vi "Accept UDP command logic.vi"(9 "Msg in":T1, 10 "MC IP":string, 11 "Msg in 2":T1) -> (2 "Boolean":bool, 3 "data":string)   [LabVIEW 2020, in "UDPComm.lvlib"]
uses:
  UDPComm.lvlib
  UDP_FGV.ctl
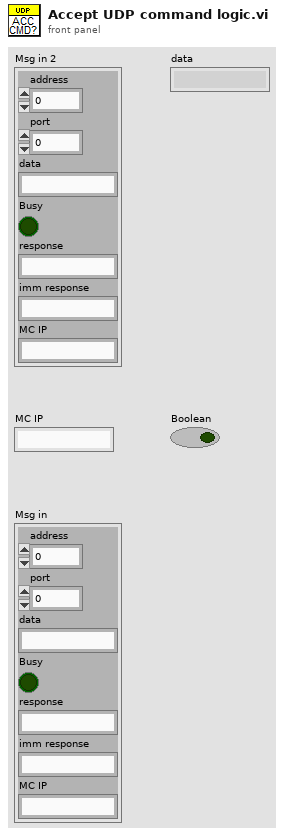
[diagram p1: front panel]
types:
  T1 = typedef "UDP_FGV.ctl" = cluster{"address":u32, "port":u16, "data":string, "Busy":bool, "response":string, "imm response":string, "MC IP":string}
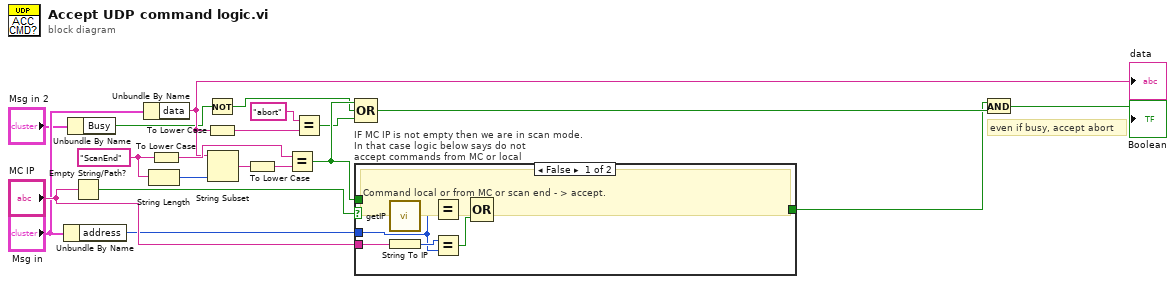
[diagram p0: block diagram]
diagram:
  w16 = "ScanEnd" ("Command")
  # "even if busy, accept abort"
  n1 = Unbundle By Name("Msg in") -> ("address"=w4:u32)
  n2 = Unbundle By Name("Msg in 2") -> ("Busy"=w9:bool)
  n3 = Empty String/Path?(string/path="MC IP") -> (empty?=w3:bool)
  n4 = Unbundle By Name("Msg in") -> ("data"=w15:string)
  "data" <- w15
  n5 = String Length(string=w16) -> (length=w14:i32)
  n6 = To Lower Case(string=w16) -> (all lower case string=w17:string)
  n7 = Not(x=w9) -> (.not. x?=w11:bool)
  n8 = To Lower Case(string=w15) -> (all lower case string=w13:string)
  n9 = String Subset(string=w15, length (rest)=w14) -> (substring=w19:string)  [unwired: 1 in]
  n10 = To Lower Case(string=w19) -> (all lower case string=w18:string)
  n11 = Equal?(x=w17, y=w18) -> (x = y?=w20:bool)
  n12 = Equal?(x="abort", y=w13) -> (x = y?=w10:bool)
  n13 = Compound Arithmetic op=OR(w20, w11, w10) -> (w12:bool)
  n14 = case "IF MC IP is not empty then we are in scan mode. In that case logic below says do not\naccept commands from MC or local" shown="False" w3 {
    selector: w3 -> [_ w29]
    tunnel: "MC IP" -> [w26 _]
    tunnel: w4 -> [w22 _]
    tunnel: [w24 w29] -> w7
    tunnel: w20 -> [w21 _]
    frame False {
      # "Command local or from MC or scan end - > accept."
      n15 = call "getIP.vi"() -> ("net address matching DB subnet"=w23:u32)  [unwired: 5 in, 3 out]
      n16 = String To IP(1:w26) -> (0:w28:u32)
      n17 = Equal?(x=w23, y=w22) -> (x = y?=w25:bool)
      n18 = Equal?(x=w28, y=w22) -> (x = y?=w27:bool)
      n19 = Compound Arithmetic op=OR(w21, w25, w27) -> (w24:bool)
    }
    frame True {
      # "MC empty. not in scan mode. accept command"
    }
  }
  n20 = And(x=w7, y=w12) -> (x .and. y?=→"Boolean":bool)
